vi "Send Message.vi"(4 "timeout in ms (100)":i32=100, 6 "ID":string, 8 "error in (no error)":errorcluster, 9 "Data":variant, 10 "Command":string, 11 "RemoteControl in":refnum<class "RemoteControl.lvclass">) -> (0 "error out":errorcluster, 2 "ACK":string, 3 "RemoteControl out":refnum<class "RemoteControl.lvclass">)   [LabVIEW 2019, in "RemoteControl.lvclass"]
uses:
  RemoteControl.lvclass
  Typedefs/Message--Cluster.ctl
  Private/RemoteControlGlobal.vi
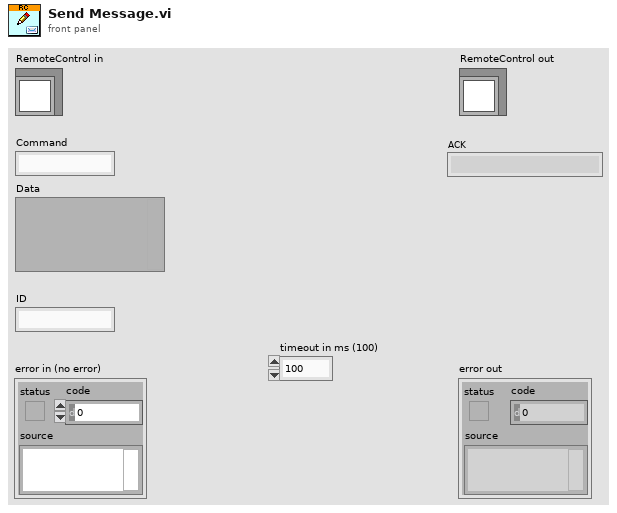
[diagram p1: front panel]
types:
  T1 = typedef "RemoteControl.lvclass/Message--Cluster.ctl" = cluster{"Command":string, "Data":variant, "ID":string}
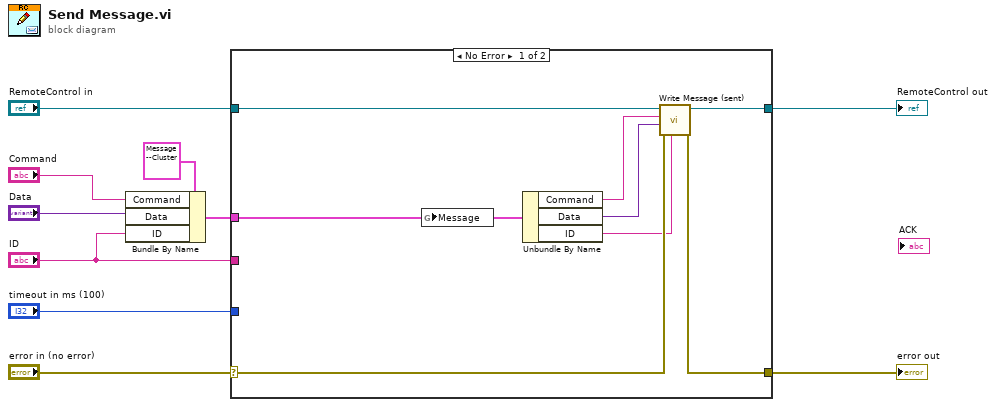
[diagram p0: block diagram]
diagram:
  n1 = Bundle By Name(cluster=T1 {"Command"="", "Data"=variant, "ID"=""} ("Message"), "Command"="Command", "Data"="Data", "ID"="ID") -> (w5:T1)
  n2 = case shown="No Error" "error in (no error)" {
    selector: "error in (no error)" -> [w16 w20]
    tunnel: [w15 w20] -> w9
    tunnel: [w18 w19] -> w7
    tunnel: "RemoteControl in" -> [w17 w19]
    tunnel: w5 -> [w14 _]
    tunnel: "timeout in ms (100)" -> [_ _]
    tunnel: "ID" -> [_ _]
    frame No Error {
      n3 = global write "RemoteControlGlobal.vi" "Message"(w14) -> ()
      n4 = Unbundle By Name(w14) -> ("Command"=w13:string, "Data"=w12:variant, "ID"=w11:string)
      n5 = call "Write Message (sent).vi"("ID (sent)"=w11, "error in (no error)"=w16, "Data (sent)"=w12, "Command (sent)"=w13, "RemoteControl in"=w17) -> ("error out"=w15:errorcluster, "RemoteControl out"=w18:refnum<class "RemoteControl.lvclass">)  [unwired: 5 in]
    }
    frame Error {
    }
  }
  "error out" <- w9
  "RemoteControl out" <- w7
